vi "ReadCurrentTriple.vi"(8 "error in (no error)":errorcluster, 11 "VISA resource name":refnum<visa-resource-name>) -> (0 "error out":errorcluster, 2 "Current":dbl[](array[numeric]), 3 "VISA resource name out":refnum<visa-resource-name>)   [LabVIEW 2012]
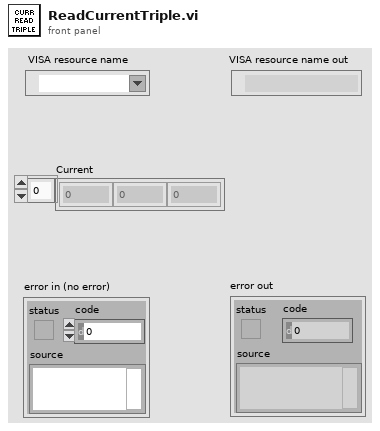
[diagram p1: front panel]
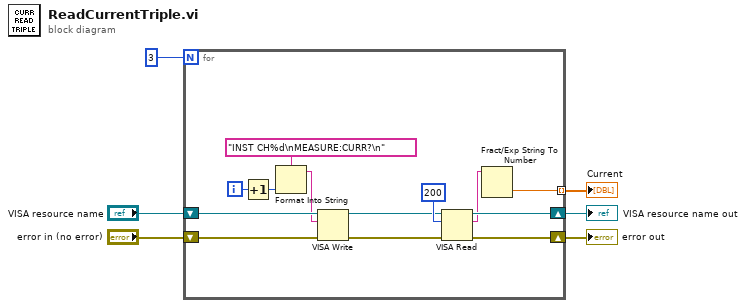
[diagram p0: block diagram]
diagram:
  n1 = for {
    N: 3 -> [_]
    shift-right: [w19] -> w1
    shift-left: "VISA resource name" -> [w16]
    shift-right: [w18] -> w2
    shift-left: "error in (no error)" -> [w15]
    tunnel: [w11] -> w3 mode=indexing
    i -> [w10]
    n2 = Increment(x=w10) -> (x+1=w9:i32)
    n3 = Format Into String(format string="INST CH%d\nMEASURE:CURR?\n", w9) -> (resulting string=w14:string)  [unwired: 2 in, 1 out]
    n4 = VISA Write(VISA resource name=w16, write buffer=w14, error in (no error)=w15) -> (VISA resource name out=w8:refnum<visa-resource-name>, error out=w7:errorcluster)  [unwired: 1 out]
    n5 = VISA Read(VISA resource name=w8, byte count=u32 200, error in (no error)=w7) -> (VISA resource name out=w19:refnum<visa-resource-name>, read buffer=w12:string, error out=w18:errorcluster)  [unwired: 1 out]
    n6 = Fract/Exp String To Number(string=w12) -> (number=w11:dbl)  [unwired: 3 in, 1 out]
  }
  "VISA resource name out" <- w1
  "error out" <- w2
  "Current" <- w3
